vi "VRESET to 2_75V.vi"(8 "error in":errorcluster) -> (0 "error out":errorcluster, 2 "Pass/Fail":bool)   [LabVIEW 2009]
uses:
  <vilib>/Instr/_visa.llb/VISA Configure Serial Port (Instr).vi
  Global/Global 1.vi
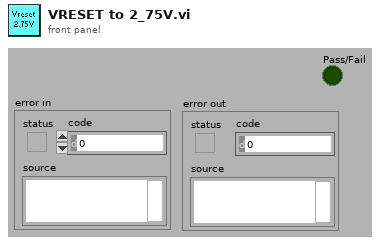
[diagram p1: front panel]
types:
  T1 = enum16{"lock key", "POwer OFF", "Power ON", "SET Volt and Current"}
  T2 = cluster{"VHEATFUSENOLOADMIN":string, "VHEATFUSELOADMAX":string, "VOVERRIDEDIODEMIN":string, "TDIFFMAX":string, "MEASFREQMAX":string, "MEASFREQMIN":string, "VOVER":string, "VMIDDLE":string, "VUNDER":string, "VNORESET":string, "VRESET":string, "WAITPING":string, "LRFID":string, "RFIDUID":string, "EXTEESIZE":string, "LCUTYPE":string, "LCUSUBTYPE":string, "TEVN":string, "BOOTVER":string, "APPVER":string, "ISLEEPMAX":string, "TSLEEP":string, "APPWAIT":string, "DBWAIT":string}
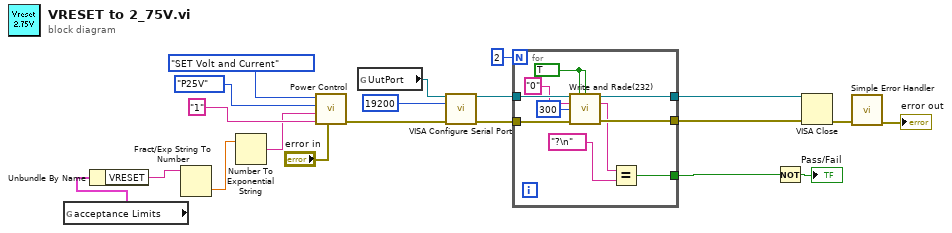
[diagram p0: block diagram]
diagram:
  n1 = global read "Global 1.vi" "acceptance Limits"() -> (w3:T2)
  n2 = Unbundle By Name(w3) -> ("VRESET"=w2:string)
  n3 = Fract/Exp String To Number(string=w2) -> (number=w1:dbl)  [unwired: 4 out]
  n4 = Number To Exponential String(number=w1) -> (E-format string=w10:string)  [unwired: 3 out]
  n5 = call "Power Control.vi"("error in"="error in", "Current"="1", "Voltage"=w10, "Channel"=enum16{"P6V", "P25V", "N25V"}."P25V", "command"=T1."SET Volt and Current") -> ("error out"=w9:errorcluster)  [unwired: 6 out]
  n6 = global read "Global 1.vi" "UutPort"() -> (w20:refnum<visa-resource-name>)
  n7 = call-poly "VISA Configure Serial Port"("VISA resource name"=w20, "baud rate (9600)"=u32 19200, "error in (no error)"=w9) -> ("VISA resource name out"=w19:refnum<visa-resource-name>, "error out"=w7:errorcluster)  [unwired: 3 in, 8 out]
  n8 = for {
    N: 2 -> [_]
    tunnel: w19 -> [w30]
    tunnel: [w29] -> w15
    tunnel: [w28] -> w14
    tunnel: w7 -> [w27]
    tunnel: [w26] -> w6
    w22 = TRUE ("write")
    n9 = call "Write and Rade(232).vi"("VISA resource name in"=w30, "write"=w22, "read"=w22, "string to write"="0", "ms delay"=u32 300, "error in"=w27) -> ("VISA resource name out"=w28:refnum<visa-resource-name>, "read string"=w23:string, "error out"=w29:errorcluster)  [unwired: 2 in, 5 out]
    n10 = Equal?(x=w23, y="?\n") -> (x = y?=w26:bool)
  }
  n11 = Not(x=w6) -> (.not. x?=→"Pass/Fail":bool)
  n12 = VISA Close(VISA resource name=w14, error in (no error)=w15) -> (error out=w17:errorcluster)
  n13 = call <vilib>:"Simple Error Handler.vi"("error in (no error)"=w17) -> ("error out"=→"error out":errorcluster)  [unwired: 1 in, 7 out]
